vi "Dependent Hierarchy.vi"() -> ()   [LabVIEW 2017, in "CL_G3_VIComponentBuilder.lvlib" / "Build Analyzer.lvclass"]
doc: "An example application that \n1. Displays the dependencies of a given export in a tree structure.\n2. Analyzes select exports of the working set and returns a build order."
uses:
  Build Analyzer.lvclass
  Exports/Exports/Export.lvclass
  Components/Component.lvclass/Component.ctl
  Build Analyzer.lvclass/Build Analyzer.ctl
  Exports/Exports/Export.lvclass/Export.ctl
  Components/Accessors/Read Component Operations Errors.vi
  Exports/Exports/Accessors/Read Product Name.vi
  Accessors/Read Product Name - Unique Name.vi
  Accessors/Write Bubble Up Working Set.vi
  Components/Component.lvclass
panel:
  in  "Build Type":T1(ring)
  out "Ordered Exports":refnum<class "Export.lvclass">[](array[class])
  out "Build Order":string[](array[string])
  in  "Select all":bool
  in  "Clear":bool
  in  "Tree":string(tree)
  in  "Analyze":bool
  in  "Components to build":u16[](array[ring]) items=["agilent 3631a", "agilent 5313x", "agilent e4980 driver", "airjet", "ap27xx", "apx5xx", "audio driver palette installer", "cbt", "class copier", "cli cache generation", "clive", "cmw", "component builder - nipkg - lv", "component installer - nipkg - lv", "componentinstaller", "database logging teststand api", "database logging teststand api - hack", "db utility", "digital driver palette installer", "dmm class", "dmm driver palette installer", "email text result", "email text result teststand api", "email text result teststand api - hack", "extensions for component builder - nipkg - lv", "extensions for labview atlassian api - nipkg - lv", "g3 extensions for labview atlassian api", "g3 teststand customizations", "hsdio serial interface", "hsdio teststand api", "hsdio teststand api - hack", "i2c digital waveform", "instek psmx", "instrument class", "instrument driver palette installer", "iteration tools", "iteration tools teststand api", "iteration tools teststand api - hack", "keithley 2000", "keithley 24xx", "keithley 26xx", "keysight cx3300 vendor driver", "labview atlassian api", "labview atlassian api - nipkg - lv", "labview auto documentation", "labview auto documentation - nipkg - lv", "labview auto documentation applicaitons - nipkg - lv", "labview auto documentation applications", "msaval build process extensions - nipkg", "ni dc power", "ni-dmm", "ni-dsa", "ni-scope", "power supply", "power supply driver palette installer", "power supply- agilent e3648a", "promira", "reusables", "reuseables - nipkg", "rf driver palette installer", "rohde & schwarz fsl vendor driver", "rssmb 100a", "scope driver palette installer", "sensata tmu", "signal generator driver palette installer", "silicon delta", "tektronix afg2k 3k", "tektronix rsa 6100 driver", "tektronix scope", "thermal driver palette installer", "val resources"]
  in  "stop":bool
  in  "Menu Ring":u16(ring) items=["agilent 3631a", "agilent 5313x", "agilent e4980 driver", "airjet", "ap27xx", "apx5xx", "audio driver palette installer", "cbt", "class copier", "cli cache generation", "clive", "cmw", "component builder - nipkg - lv", "component installer - nipkg - lv", "componentinstaller", "database logging teststand api", "database logging teststand api - hack", "db utility", "digital driver palette installer", "dmm class", "dmm driver palette installer", "email text result", "email text result teststand api", "email text result teststand api - hack", "extensions for component builder - nipkg - lv", "extensions for labview atlassian api - nipkg - lv", "g3 extensions for labview atlassian api", "g3 teststand customizations", "hsdio serial interface", "hsdio teststand api", "hsdio teststand api - hack", "i2c digital waveform", "instek psmx", "instrument class", "instrument driver palette installer", "iteration tools", "iteration tools teststand api", "iteration tools teststand api - hack", "keithley 2000", "keithley 24xx", "keithley 26xx", "keysight cx3300 vendor driver", "labview atlassian api", "labview atlassian api - nipkg - lv", "labview auto documentation", "labview auto documentation - nipkg - lv", "labview auto documentation applicaitons - nipkg - lv", "labview auto documentation applications", "msaval build process extensions - nipkg", "ni dc power", "ni-dmm", "ni-dsa", "ni-scope", "power supply", "power supply driver palette installer", "power supply- agilent e3648a", "promira", "reusables", "reuseables - nipkg", "rf driver palette installer", "rohde & schwarz fsl vendor driver", "rssmb 100a", "scope driver palette installer", "sensata tmu", "signal generator driver palette installer", "silicon delta", "tektronix afg2k 3k", "tektronix rsa 6100 driver", "tektronix scope", "thermal driver palette installer", "val resources"]
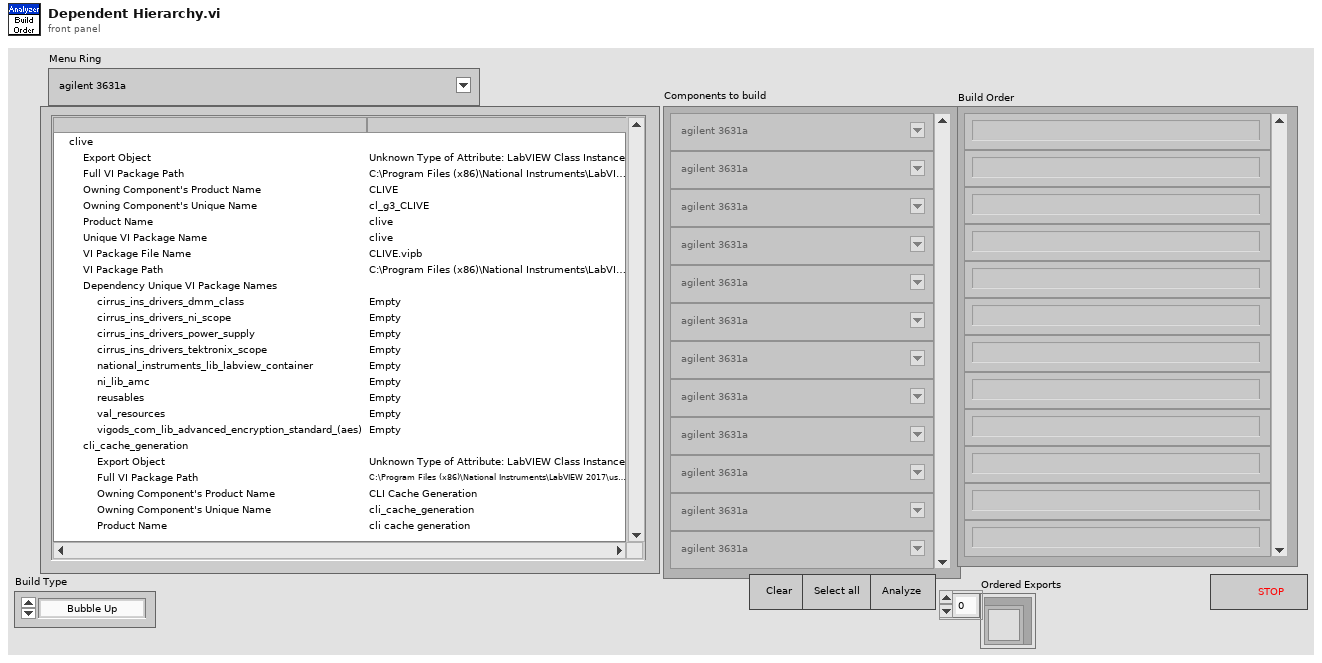
[diagram p1: front panel]
types:
  T1 = enum16{"Bubble Up", "Build Dependencies", "Build Selected Only"}
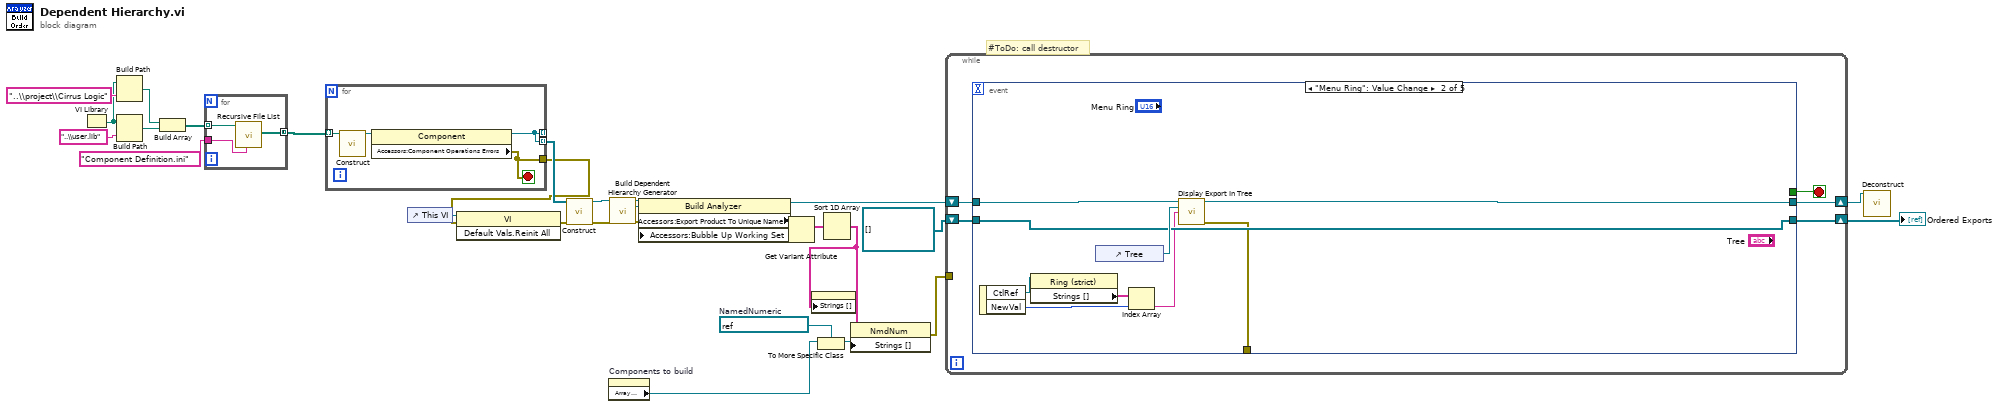
[diagram p0: block diagram]
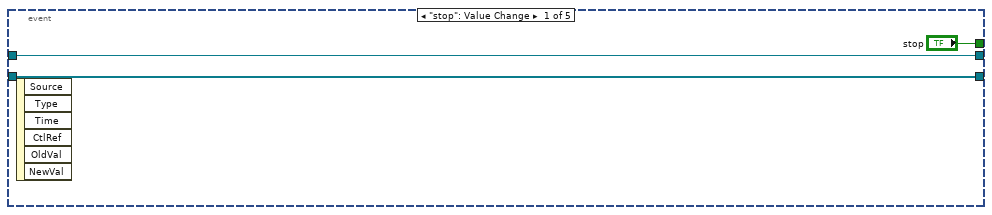
[diagram p2: hidden frame]
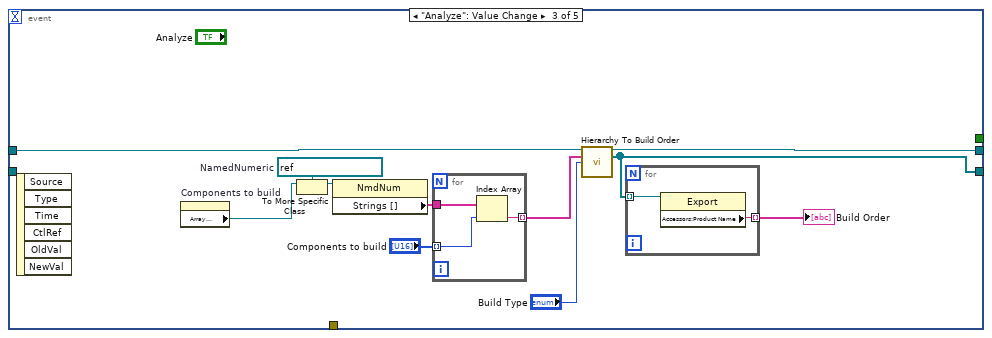
[diagram p3: hidden frame]
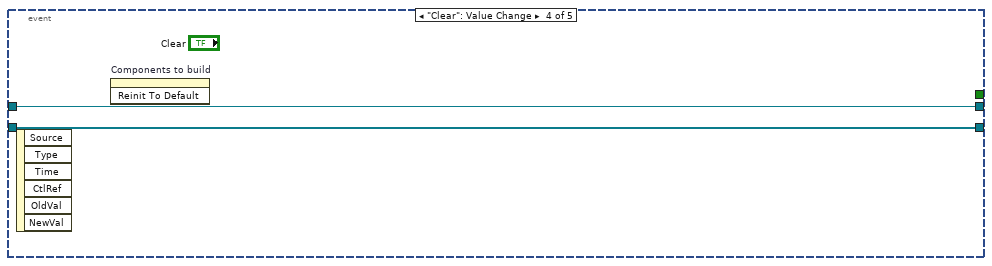
[diagram p4: hidden frame]
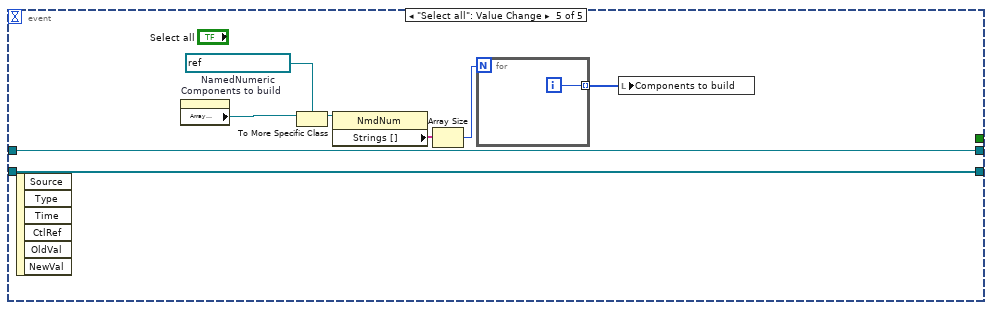
[diagram p5: hidden frame]
diagram:
  w22 = refnum<vi> refnum  # NamedNumeric
  # "#ToDo: call destructor"
  n1 = VI Library() -> (path=w24:path)
  n2 = Build Path(base path=w24, name or relative path="..\\project\\Cirrus Logic") -> (appended path=w25:path)
  n3 = Build Path(base path=w24, name or relative path="..\\user.lib") -> (appended path=w26:path)
  n4 = Build Array(w25, w26) -> (w14:path[])
  n5 = for {
    tunnel: w14 -> [w31] mode=indexing
    tunnel: [w30] -> w3 mode=concatenating
    tunnel: "Component Definition.ini" ("pattern") -> [w29]
    n6 = call <vilib>:"Recursive File List.vi"("pattern"=w29, "Folder Path"=w31) -> ("All Files in Dir"=w30:path[])  [unwired: 5 in, 4 out]
  }
  n7 = for {
    tunnel: w3 -> [w34] mode=indexing
    tunnel: [w32] -> _ mode=indexing
    tunnel: [w33] -> w1
    tunnel: [w32] -> w2 mode=indexing
    stop <- w33 stop-if-true
    n8 = call "Construct.vi"("Component Config File"=w34) -> ("Component"=w35:refnum<class "Component.lvclass">)  [unwired: 14 in]
    n9 = property class="Component"(reference=w35) -> (reference out=w32:refnum<class "Component.lvclass">, "Accessors:Component Operations Errors"=w33:errorcluster)  [unwired: 1 in, 1 out]
  }
  n10 = control-ref of="This VI"() -> (w18:refnum<vi>)
  n11 = invoke class="VI" method="Default Vals.Reinit All"(reference=w18, error in=w1) -> (error out=w15:errorcluster)  [unwired: 1 in, 2 out]
  n12 = call "Construct.vi"("Components"=w2, "error in (no error)"=w15) -> ("Build Analyzer"=w8:refnum<class "Build Analyzer.lvclass">, "error out"=w5:errorcluster)  [unwired: 12 in]
  n13 = property on="Components to build" class="Arr (strict)"() -> ("Array Element"=w20:refnum<vi>)  [unwired: 2 in, 2 out]
  n14 = call "Build Dependent Hierarchy Generator.vi"("Build Analyzer in"=w8, "error in (no error)"=w5) -> ("dup Build Analyze"=w7:refnum<class "Build Analyzer.lvclass">, "Bubbe Up Working Set"=w6:refnum<data-value>, "error out"=w4:errorcluster)  [unwired: 11 in]
  n15 = property class="Build Analyzer"(reference=w7, error in=w4, "Accessors:Bubble Up Working Set"=w6) -> (reference out=w9:refnum<class "Build Analyzer.lvclass">, "Accessors:Export Product To Unique Name"=w12:variant)  [unwired: 1 out]
  n16 = Get Variant Attribute(Variant=w12) -> (names=w19:string[])  [unwired: 3 in, 3 out]
  n17 = To More Specific Class(target class=w22, reference=w20) -> (specific class reference=w23:refnum<vi>)  [unwired: 1 in, 1 out]
  n18 = Sort 1D Array(array=w19) -> (sorted array=w21:string[])
  n19 = property on="Menu Ring" class="Ring (strict)"("Strings []"=w21) -> ()  [unwired: 2 in, 2 out]
  n20 = property class="NmdNum"(reference=w23, "Strings []"=w21) -> (error out=w16:errorcluster)  [unwired: 1 in, 1 out]
  n21 = while {
    shift-right: [w38] -> w11
    shift-left: refnum<class "Export.lvclass">[] [] ("Ordered Exports") -> [w39]
    tunnel: w16 -> [_]
    shift-right: [w36] -> w10
    shift-left: w9 -> [w37]
    stop <- w40 stop-if-true
    n22 = event shown="[1] \"Menu Ring\": Value Change" {
      selector: _ -> [_ _ _ _ _]
      dyn-events: _ -> [_ _ _ _ _]
      timeout: _ -> [_ _ _ _ _]
      tunnel: ["stop" _ _ _ _] -> w40
      tunnel: w37 -> [w41 w44 w54 w69 w71]
      tunnel: [w42 w48 w56 w70 w78] -> w38
      tunnel: w39 -> [w42 w48 _ w70 w78]
      tunnel: [w41 w46 w55 w69 w71] -> w36
      tunnel: [_ w45 _ _ _] -> _
      event "stop": Value Change {
        n23 = event-data() -> ()  [unwired: 1 in, 6 out]
      }
      event "Menu Ring": Value Change {
        n24 = event-data() -> ("CtlRef"=w52:refnum<vi>, "NewVal"=w50:u16)  [unwired: 1 in]
        n25 = property class="Ring (strict)"(reference=w52) -> ("Strings []"=w51:string[])  [unwired: 1 in, 2 out]
        n26 = control-ref of="Tree"() -> (w49:refnum<vi>)
        n27 = Index Array(array=w51, index=w50) -> (element=w47:string)
        n28 = call "Display Export In Tree.vi"("Build Analyzer in"=w44, "Tree"=w49, "Product Name"=w47) -> ("Build Analyzer out"=w46:refnum<class "Build Analyzer.lvclass">, "error out"=w45:errorcluster)  [unwired: 11 in]
      }
      event "Analyze": Value Change {
        w63 = refnum<vi> refnum  # NamedNumeric
        n29 = event-data() -> ()  [unwired: 1 in, 6 out]
        n30 = property on="Components to build" class="Arr (strict)"() -> ("Array Element"=w61:refnum<vi>)  [unwired: 2 in, 2 out]
        n31 = To More Specific Class(target class=w63, reference=w61) -> (specific class reference=w62:refnum<vi>)  [unwired: 1 in, 1 out]
        n32 = property class="NmdNum"(reference=w62) -> ("Strings []"=w60:string[])  [unwired: 1 in, 2 out]
        n33 = for {
          tunnel: w60 -> [w68]
          tunnel: "Components to build" -> [w67] mode=indexing
          tunnel: [w66] -> w57 mode=indexing
          n34 = Index Array(array=w68, index=w67) -> (element=w66:string)
        }
        n35 = call "Hierarchy To Build Order.vi"("Build Analyzer in"=w54, "Export Product Names to build"=w57, "Build Type"="Build Type") -> ("dup Build Analyzer"=w55:refnum<class "Build Analyzer.lvclass">, "Ordered Exports"=w56:refnum<class "Export.lvclass">[])  [unwired: 10 in, 1 out]
        n36 = for {
          tunnel: w56 -> [w65] mode=indexing
          tunnel: [w64] -> w58 mode=indexing
          n37 = property class="Export"(reference=w65) -> ("Accessors:Product Name"=w64:string)  [unwired: 1 in, 2 out]
        }
        "Build Order" <- w58
      }
      event "Clear": Value Change {
        n38 = event-data() -> ()  [unwired: 1 in, 6 out]
        n39 = invoke on="Components to build" class="Arr (strict)" method="Reinit To Default"() -> ()  [unwired: 3 in, 3 out]
      }
      event "Select all": Value Change {
        w76 = refnum<vi> refnum  # NamedNumeric
        n40 = event-data() -> ()  [unwired: 1 in, 6 out]
        n41 = property on="Components to build" class="Arr (strict)"() -> ("Array Element"=w72:refnum<vi>)  [unwired: 2 in, 2 out]
        n42 = To More Specific Class(target class=w76, reference=w72) -> (specific class reference=w77:refnum<vi>)  [unwired: 1 in, 1 out]
        n43 = property class="NmdNum"(reference=w77) -> ("Strings []"=w75:string[])  [unwired: 1 in, 2 out]
        n44 = Array Size(array=w75) -> (size(s)=w74:i32)
        n45 = for {
          N: w74 -> [_]
          tunnel: [w79] -> w73 mode=indexing
          i -> [w79]
        }
        n46 = local write "Components to build"(w73) -> ()
      }
    }
  }
  "Ordered Exports" <- w11
  n47 = call "Deconstruct.vi"("Build Analyzer"=w10) -> ()  [unwired: 14 in, 1 out]
